vi "Fluigent_Pressure_Fluctuation.vi"() -> ()   [LabVIEW 2020]
uses:
  <vilib>/Utility/error.llb/DialogType.ctl
  <vilib>/DAQmx/write.llb/DAQmx Write (Analog DBL 1Chan 1Samp).vi
  <vilib>/DAQmx/read.llb/DAQmx Read (Analog 1D Wfm NChan NSamp).vi
  <vilib>/DAQmx/create/channels.llb/DAQmx Create Channel (AI-Voltage-Basic).vi
  <vilib>/DAQmx/configure/timing.llb/DAQmx Timing (Sample Clock).vi
  <userlib>/Fluigent/Fluigent MFCS/FluigentMFCS_Full.llb/MFCS_EZ Detect.vi
  <userlib>/Fluigent/Fluigent MFCS/FluigentMFCS_Full.llb/MFCS_EZ Initialization.vi
  <vilib>/Waveform/WDTOps.llb/WDT Get XY Value DBL.vi
  <userlib>/Fluigent/Fluigent MFCS/FluigentMFCS_Full.llb/MFCS_EZ Read All Channels Pressure.vi
  <vilib>/DAQmx/miscellaneous.llb/DAQmx Fill In Error Info.vi
  <userlib>/Fluigent/Fluigent MFCS/FluigentMFCS_Full.llb/MFCS_EZ Close.vi
  <vilib>/measure/NI_MABase.lvlib
panel:
  in  "Index File Labels Fluigent System":string[](array[string])=["1000", "nobody", "test", "1", "1", "junk"]
  out "Analog File Name Fluigent":string="C:\\yurong\\141104_12_31_1104"
  in  "Path for files Fluigent System":path=path "C:/Users/kkg5246/Desktop/Research/Fluigent Recordings"
  in  "sampling info":cluster{"Fs":dbl, "#s":dbl}={"Fs"=100.0, "#s"=1000.0} {"Fs" format="%0.2p"}
  out "Current Voltage\n(V)":dbl
  out "Current Pressure\n(mmHg)":dbl
  out "Actual Presure":dbl[](graph)
  out "Theoretical Pressure Waveform":waveform(dbl)(graph)={"t0"=timestamp(15 s since 1904-01-01), "dt"=0.001, "Y"=[]}
  in  "Voltage Conversion Factor":dbl=100.0 caption="Voltage Conversion Factor (1 V = x mmHg)" format="%0.2f"
  in  "Duty Cycle (%)":dbl=50.0 format="%0.2f"
  in  "Offset":dbl=250.0 format="%0.2p"
  in  "Reset Signal ?":bool
  in  "Signal Type":T1(ring)
  in  "Frequency (Hz)":dbl=5.0 format="%0.2p"
  in  "Amplitude (mmHg)":dbl=0.25 format="%0.2p"
  in  "Phase":dbl format="%0.2f"
  out "phase out":dbl=180.0000000002135 format="%0.2f"
  in  "stop 2":bool
  out "Waveform Chart":waveform(dbl)(graph)
  out "x/y":dbl
  out "Pressure":dbl[](graph)=[0.00694105110600887]
  in  "Index File Labels":string[](array[string])=["1000", "nobody", "test", "1", "1", "junk"]
  out "Analog file name":string="C:\\yurong\\141104_12_31_1104"
  in  "Path for files":path=path "C:/Users/kkg5246/Desktop/Research/Pressure Recordings"
  in  "Sampling Freq":dbl=100.0 format="%0.2f"
  in  "physical channels":tag="Dev1/ai0"
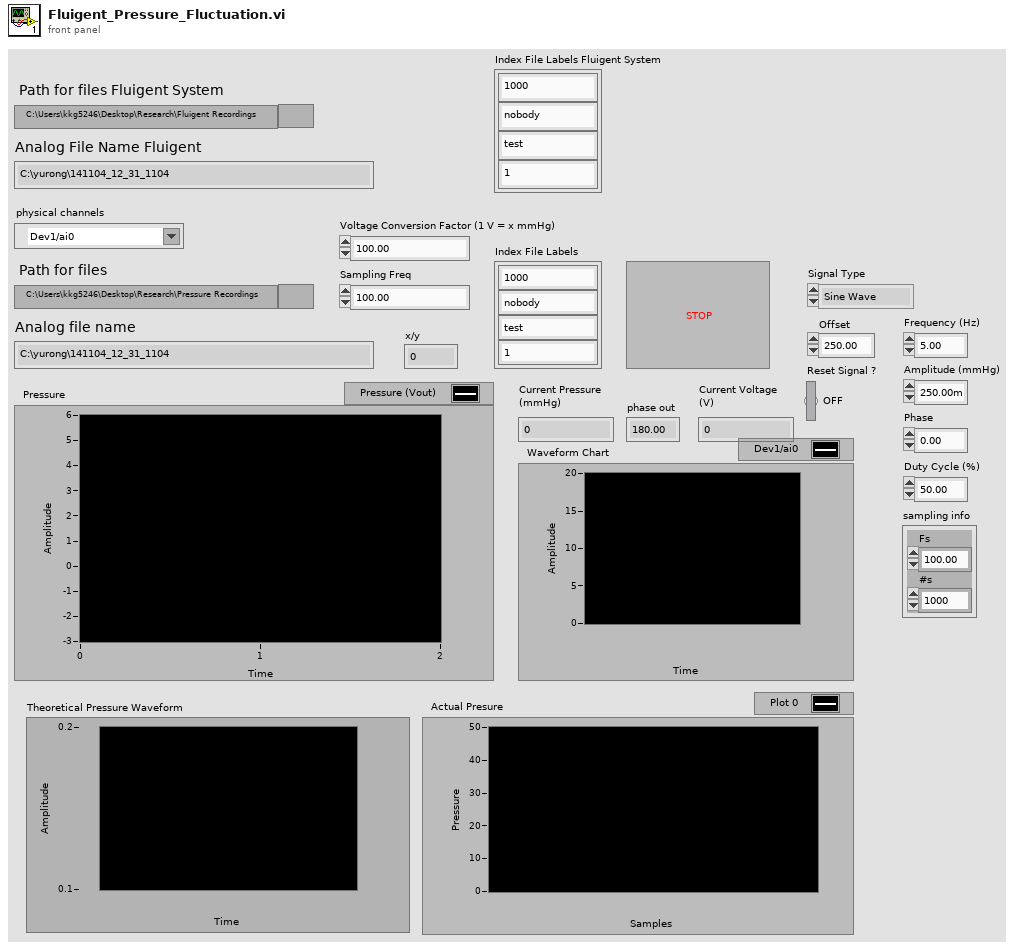
[diagram p1: front panel]
types:
  T1 = enum16{"Sine Wave", "Triangle Wave", "Square Wave", "Sawtooth Wave"}
  T2 = enum16{"open", "open or create", "create or replace", "create", "open (read-only)"}
  T3 = typedef "DialogType.ctl" = u16
  T4 = typedef "_EZmfcsSN.ctl" = u16
  T5 = typedef "_mfcs_EZ_handle.ctl" = u64
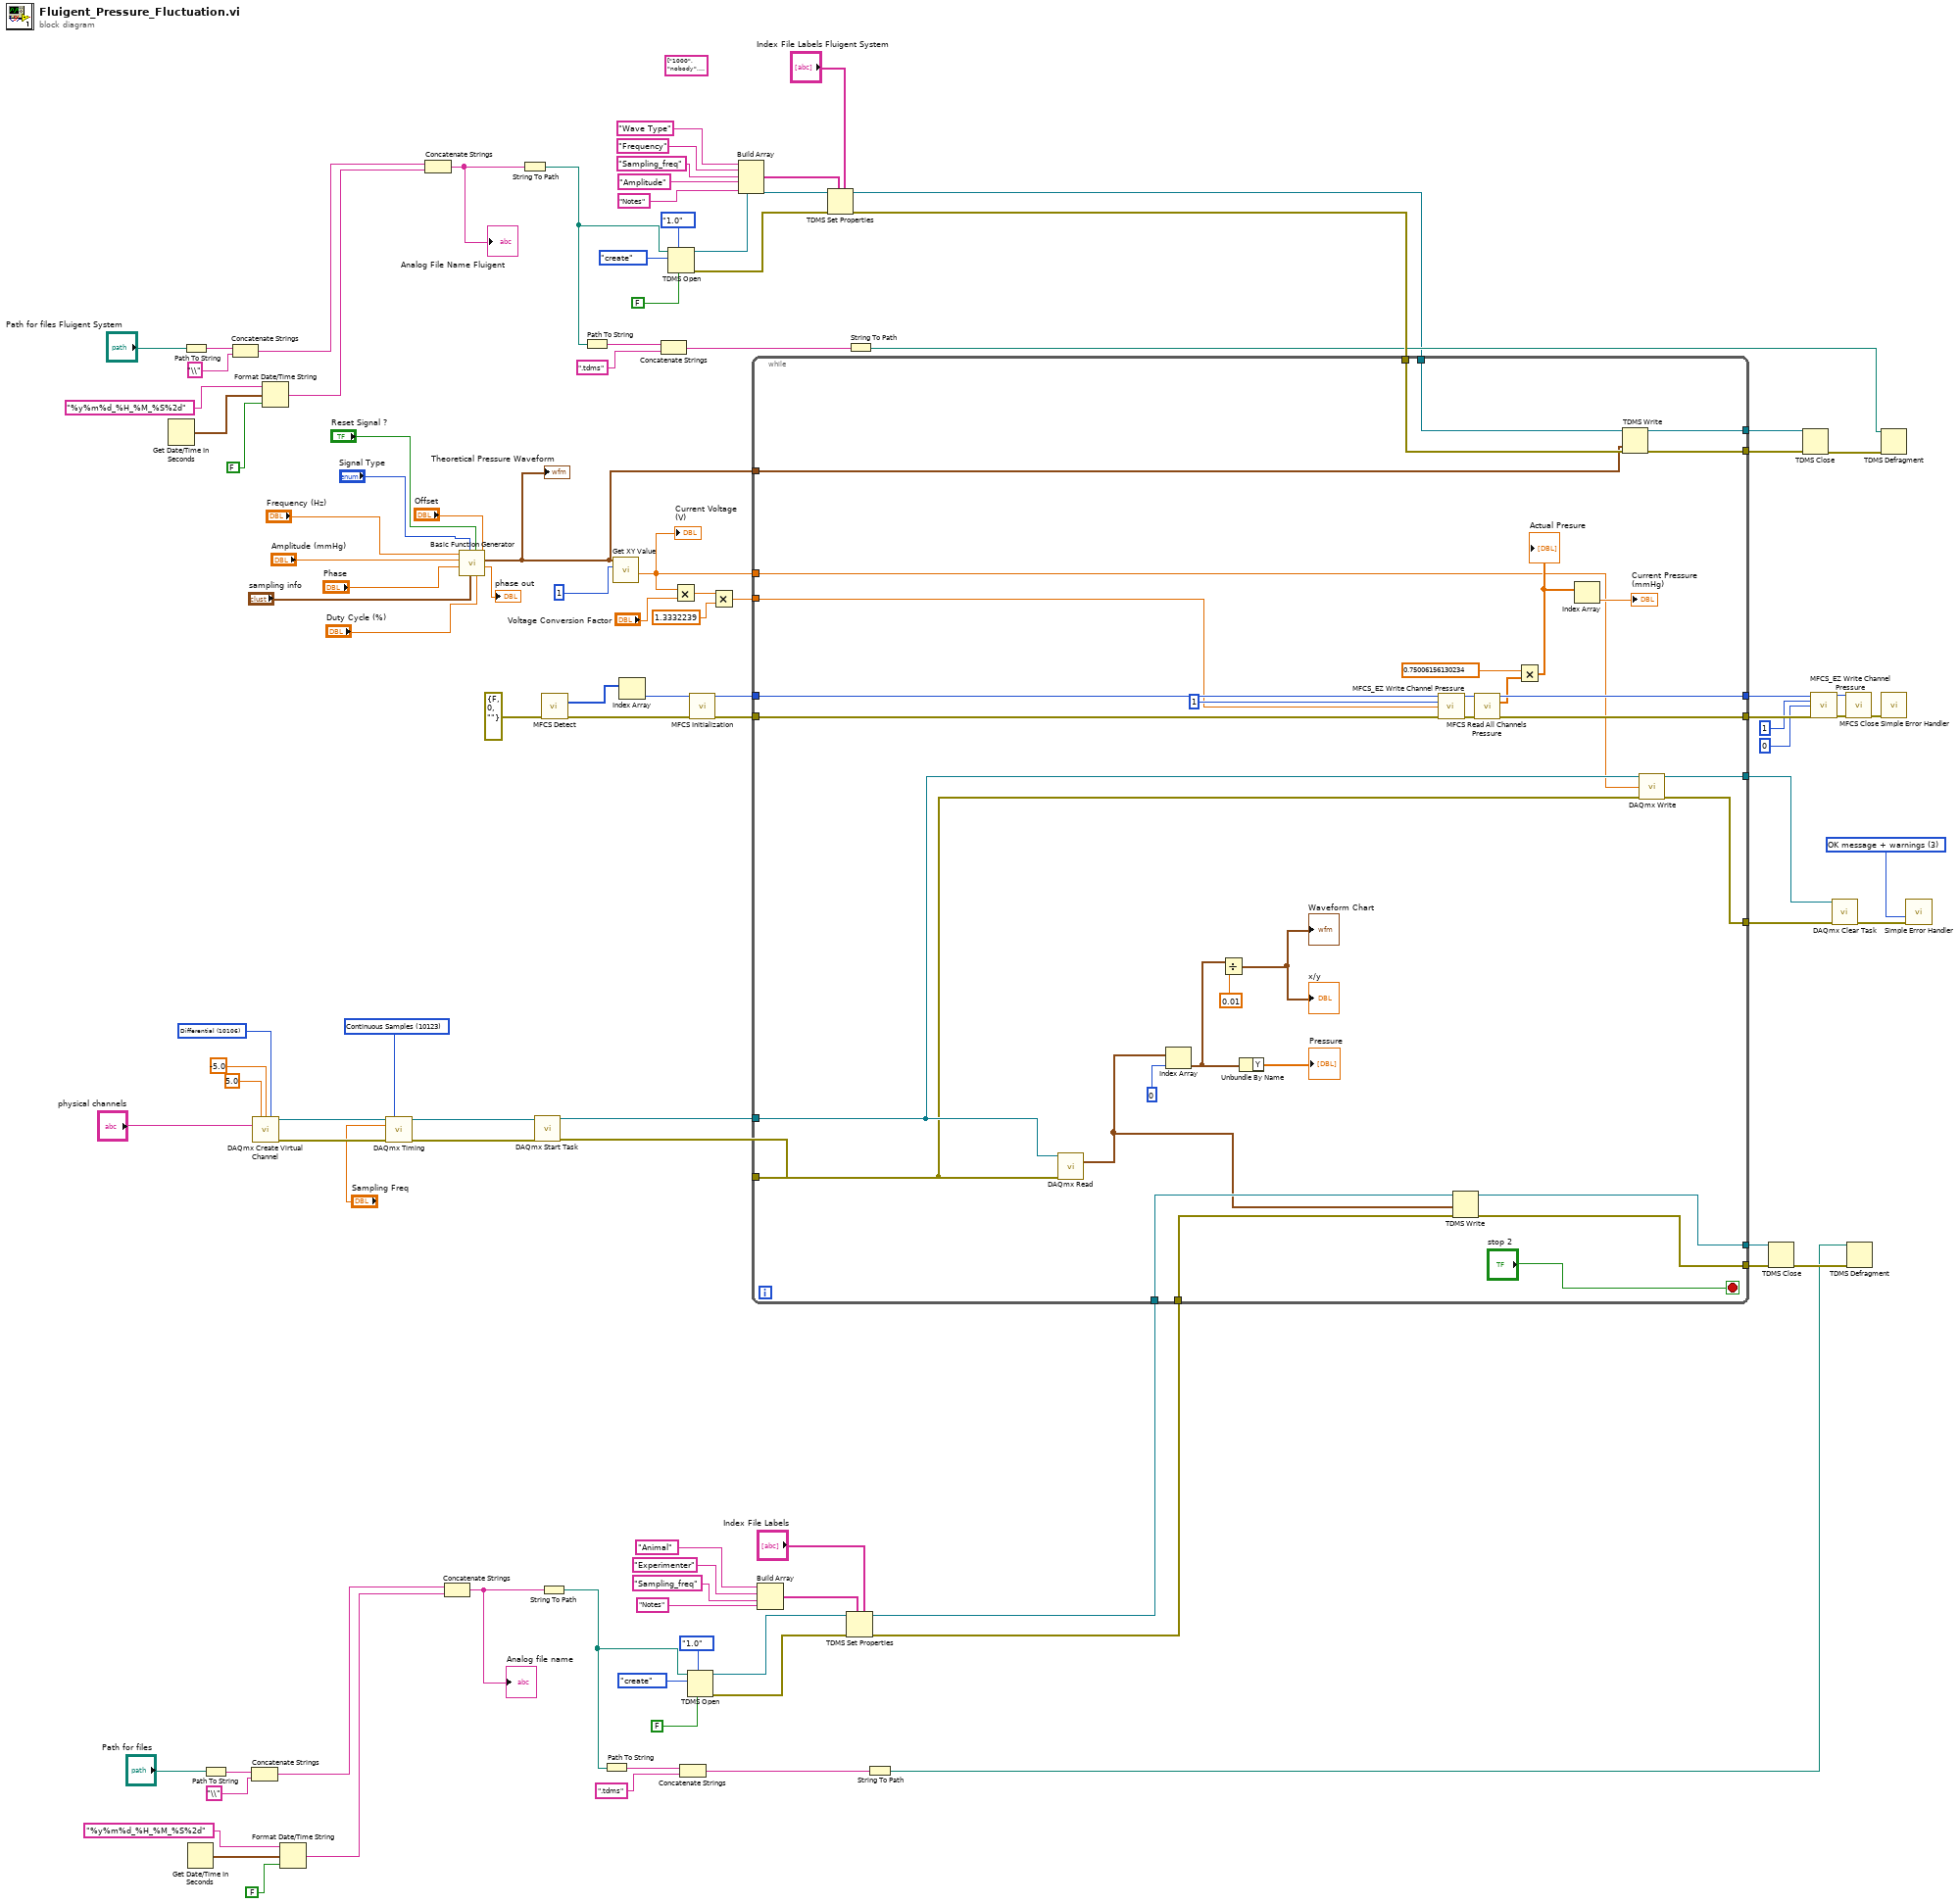
[diagram p0: block diagram]
diagram:
  (unwired) string[] ["1000", "nobody", "test", "1", "1", "junk"] ("Index File Labels Fluigent System")
  w59 = T3 3 items=["no dialog", "OK message", "continue or stop message", "OK message + warnings", "continue/stop + warnings"] ("type of dialog (OK msg:1)")
  w100 = 10106 items=["default"=-1, "RSE"=10083, "NRSE"=10078, "Differential"=10106, "Pseudodifferential"=12529] ("input terminal configuration")
  w105 = 10123 items=["Finite Samples"=10178, "Continuous Samples"=10123, "Hardware Timed Single Point"=12522] ("sample mode")
  n1 = Get Date/Time In Seconds() -> (seconds since 1Jan1904=w45:timestamp)
  n2 = Path To String(path="Path for files Fluigent System") -> (string=w27:string)
  n3 = Get Date/Time In Seconds() -> (seconds since 1Jan1904=w94:timestamp)
  n4 = Path To String(path="Path for files") -> (string=w67:string)
  n5 = Concatenate Strings(w27, "\\" ("string")) -> (w43:string)
  n6 = Concatenate Strings(w67, "\\" ("string")) -> (w92:string)
  n7 = call-poly <vilib>:"DAQmx Create Virtual Channel.vi"("maximum value"=5.0, "minimum value"=-5.0, "input terminal configuration"=w100, "physical channels"="physical channels") -> ("task out"=w106:refnum<k21>, "error out"=w104:errorcluster)  [unwired: 5 in, 5 out]
  n8 = Format Date/Time String(time format string (%c)="%y%m%d_%H_%M_%S%2d", seconds (now)=w45, UTC format=FALSE) -> (date/time string=w42:string)
  n9 = Format Date/Time String(time format string (%c)="%y%m%d_%H_%M_%S%2d", seconds (now)=w94, UTC format=FALSE) -> (date/time string=w91:string)
  n10 = call-poly <vilib>:"DAQmx Timing.vi"("task/channels in"=w106, "sample mode"=w105, "rate"="Sampling Freq", "error in"=w104) -> ("task out"=w98:refnum<k21>, "error out"=w97:errorcluster)  [unwired: 3 in, 7 out]
  n11 = Concatenate Strings(w43, w42) -> (w41:string)
  "Analog File Name Fluigent" <- w41
  n12 = Concatenate Strings(w92, w91) -> (w90:string)
  "Analog file name" <- w90
  n13 = call <vilib>:"Basic Function Generator.vi"("offset"="Offset", "square wave duty cycle (%)"="Duty Cycle (%)", "reset signal"="Reset Signal ?", "sampling info"="sampling info", "signal type"="Signal Type", "phase"="Phase", "amplitude"="Amplitude (mmHg)", "frequency"="Frequency (Hz)") -> ("phase out"=→"phase out":dbl, "signal out"=w1:waveform(dbl))  [unwired: 1 in, 1 out]
  "Theoretical Pressure Waveform" <- w1
  n14 = String To Path(string=w41) -> (path=w37:path)
  n15 = call <vilib>:"DAQmx Start Task.vi"("task/channels in"=w98, "error in"=w97) -> ("task out"=w69:refnum<k21>, "error out"=w68:errorcluster)  [unwired: 12 out]
  n16 = String To Path(string=w90) -> (path=w86:path)
  n17 = call-poly <userlib>:"MFCS Detect.vi"("error in (no error)"=errorcluster {"status"=FALSE, "code"=0, "source"=""}) -> ("[SN MFCS_EZ]"=w64:T4[], "error out"=w62:errorcluster)  [unwired: 13 in]
  n18 = Path To String(path=w37) -> (string=w36:string)
  n19 = Path To String(path=w86) -> (string=w85:string)
  n20 = call-poly <vilib>:"Get XY Value.vi"("Y position format"=1, "waveform in"=w1) -> ("Y value"=w2:dbl)  [unwired: 5 in, 4 out]
  "Current Voltage\n(V)" <- w2
  n21 = Index Array(array=w64) -> (element=w63:T4)  [unwired: 1 in]
  n22 = Concatenate Strings(w36, ".tdms" ("string")) -> (w28:string)
  n23 = TDMS Open(6:FALSE ("disable buffering? (T)"), 7:enum16{"1.0", "2.0"}."1.0" ("file format version (2.0)"), 10:T2."create" ("operation (0:open)"), 11:w37) -> (0:w34:errorcluster, 3:w25:refnum<k34>)  [unwired: 3 in]
  n24 = Multiply(x=w2, y="Voltage Conversion Factor") -> (x*y=w15:dbl)
  n25 = Concatenate Strings(w85, ".tdms" ("string")) -> (w75:string)
  n26 = TDMS Open(6:FALSE ("disable buffering? (T)"), 7:enum16{"1.0", "2.0"}."1.0" ("file format version (2.0)"), 10:T2."create" ("operation (0:open)"), 11:w86) -> (0:w83:errorcluster, 3:w65:refnum<k34>)  [unwired: 3 in]
  n27 = call-poly <userlib>:"MFCS Initialization.vi"("SN MFCS_EZ"=w63, "error in (no error)"=w62) -> ("MFCS_EZ_out"=w54:T5, "error out"=w52:errorcluster)  [unwired: 10 in, 2 out]
  n28 = Multiply(x=w15, y=1.3332239) -> (x*y=w3:dbl)
  n29 = Build Array "Build Array"("Wave Type", "Frequency", "Sampling_freq", "Amplitude", "Notes") -> (w29:string[])
  n30 = Build Array "Build Array"("Animal", "Experimenter", "Sampling_freq", "Notes") -> (w77:string[])
  n31 = TDMS Set Properties(5:"Index File Labels Fluigent System", 7:w29, 8:w34, 11:w25) -> (0:w23:errorcluster, 3:w19:refnum<k34>)  [unwired: 4 out]
  n32 = TDMS Set Properties(5:"Index File Labels", 7:w77, 8:w83, 11:w65) -> (0:w71:errorcluster, 3:w70:refnum<k34>)  [unwired: 4 out]
  n33 = while {
    tunnel: [w133] -> w73
    tunnel: [w132] -> w72
    tunnel: w71 -> [w131]
    tunnel: w70 -> [w130]
    tunnel: w69 -> [w128]
    tunnel: w68 -> [w122]
    tunnel: [w127] -> w60
    tunnel: w54 -> [w123]
    tunnel: [w121] -> w53
    tunnel: w52 -> [w120]
    tunnel: [w119] -> w51
    tunnel: [w118] -> w48
    tunnel: w23 -> [w113]
    tunnel: [w112] -> w21
    tunnel: w19 -> [w111]
    tunnel: [w110] -> w18
    tunnel: w3 -> [w109]
    tunnel: w2 -> [w108]
    tunnel: w1 -> [w107]
    stop <- "stop 2" stop-if-true
    n34 = call-poly <vilib>:"DAQmx Read.vi"("task/channels in"=w128, "error in"=w122) -> ("data"=w129:waveform(dbl)[])  [unwired: 1 in, 12 out]
    n35 = Index Array "Index Array"(array=w129, index=0 ("index (row)")) -> (element=w135:waveform(dbl))
    n36 = Divide(x=w135, y=0.01) -> (x/y=→"x/y" →"Waveform Chart":waveform(dbl))
    n37 = Unbundle By Name(w135) -> ("Y"=→"Pressure":dbl[])
    n38 = call <userlib>:"MFCS_EZ Write Channel Pressure.vi"("MFCS_EZ"=w123, "Channel Number (default=1)"=1, "Pressure (mBar)"=w109, "error in (no error)"=w120) -> ("MFCS_EZ out"=w125:T5, "error out"=w126:errorcluster)  [unwired: 10 in]
    n39 = TDMS Write(0:w130, 9:w129, 11:w131) -> (4:w132:refnum<k34>, 15:w133:errorcluster)  [unwired: 3 in, 2 out]
    n40 = call-poly <userlib>:"MFCS Read All Channels Pressure.vi"("MFCS_EZ"=w125, "error in (no error)"=w126) -> ("MFCS_EZ out"=w118:T5, "All Channels Pressure"=w117:dbl[], "error out"=w119:errorcluster)  [unwired: 11 in]
    n41 = Multiply(x=0.75006156130234, y=w117) -> (x*y=w115:dbl[])
    "Actual Presure" <- w115
    n42 = Index Array(array=w115) -> (element=→"Current Pressure\n(mmHg)":dbl)  [unwired: 1 in]
    n43 = TDMS Write(0:w111, 9:w107, 11:w113) -> (4:w110:refnum<k34>, 15:w112:errorcluster)  [unwired: 3 in, 2 out]
    n44 = call-poly <vilib>:"DAQmx Write.vi"("task/channels in"=w128, "data"=w108, "error in"=w122) -> ("task out"=w127:refnum<k21>, "error out"=w121:errorcluster)  [unwired: 10 in, 1 out]
  }
  n45 = String To Path(string=w28) -> (path=w20:path)
  n46 = String To Path(string=w75) -> (path=w74:path)
  n47 = TDMS Close(8:w73, 11:w72) -> (0:w76:errorcluster)  [unwired: 1 out]
  n48 = TDMS Close(8:w21, 11:w18) -> (0:w22:errorcluster)  [unwired: 1 out]
  n49 = call <userlib>:"MFCS_EZ Write Channel Pressure.vi"("MFCS_EZ"=w48, "Channel Number (default=1)"=1, "Pressure (mBar)"=0, "error in (no error)"=w51) -> ("MFCS_EZ out"=w55:T5, "error out"=w56:errorcluster)  [unwired: 10 in]
  n50 = call <vilib>:"DAQmx Clear Task.vi"("task in"=w60, "error in"=w53) -> ("error out"=w58:errorcluster)  [unwired: 13 in]
  n51 = call-poly <userlib>:"MFCS Close.vi"("MFCS_EZ"=w55, "error in (no error)"=w56) -> ("error out"=w57:errorcluster)  [unwired: 13 in]
  n52 = TDMS Defragment(4:w76, 7:w74) -> ()  [unwired: 1 out]
  n53 = TDMS Defragment(4:w22, 7:w20) -> ()  [unwired: 1 out]
  n54 = call <vilib>:"Simple Error Handler.vi"("error in (no error)"=w57) -> ()  [unwired: 4 in, 5 out]
  n55 = call <vilib>:"Simple Error Handler.vi"("type of dialog (OK msg:1)"=w59, "error in (no error)"=w58) -> ()  [unwired: 3 in, 5 out]
